vi "Aspect Ratio Score.vi"(10 "Height":dbl, 11 "Width":dbl) -> (3 "Score":dbl)   [LabVIEW 2013]
doc: "Compare the ratio of the rectangle to that of the expected target. Score is in percent.\n\nSince inputs are particle measurements, the diagram doesn't expect to receive zero or negative values for either input."
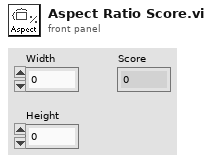
[diagram p1: front panel]
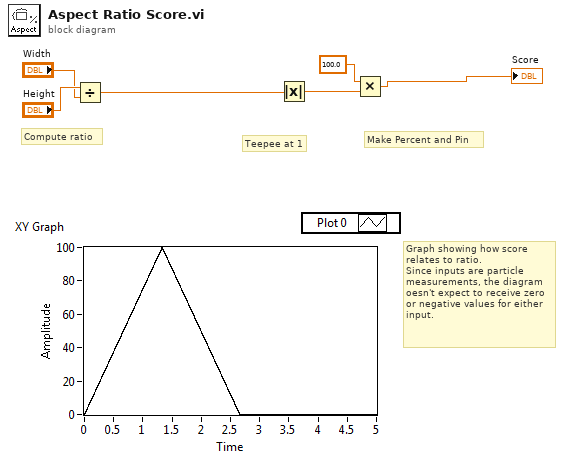
[diagram p0: block diagram]
diagram:
  # "Graph showing how score\nrelates to ratio.\nSince inputs are particle\nmeasurements, the diagram\noesn't expect to receive zero\nor negative values for either\ninput."
  # "Make Percent and Pin"
  # "Teepee at 1"
  # "Compute ratio"
  n1 = Divide(x="Height", y="Width") -> (x/y=w2:dbl)
  n2 = Absolute Value(x=w2) -> (abs(x)=w6:dbl)
  n3 = Multiply(x=100.0 ("x/y"), y=w6) -> (x*y=→"Score":dbl)
